vi "Solve General Linear Equations with SVD (DBL).vi"(8 "iteration":i32=2, 9 "relative tolerance":dbl, 10 "Known Vector":dbl[](array[numeric]), 11 "Input Matrix":T1) -> (0 "error":i32, 3 "Solution Vector":dbl[](array[numeric]))   [LabVIEW 2010, in "NI_AALPro.lvlib"]
uses:
  NI_AALPro.lvlib
  RealMatrix.ctl
  Real SVD Decomposition.vi
  Real Transpose Matrix.vi
  A x Vector.vi
  NI_AALBase.lvlib
  NI_Matrix.lvlib
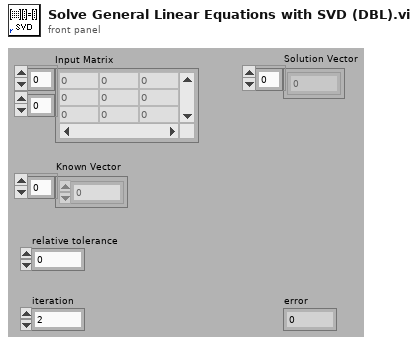
[diagram p1: front panel]
types:
  T1 = typedef "NI_Matrix.lvlib/RealMatrix.ctl" = dbl[][]
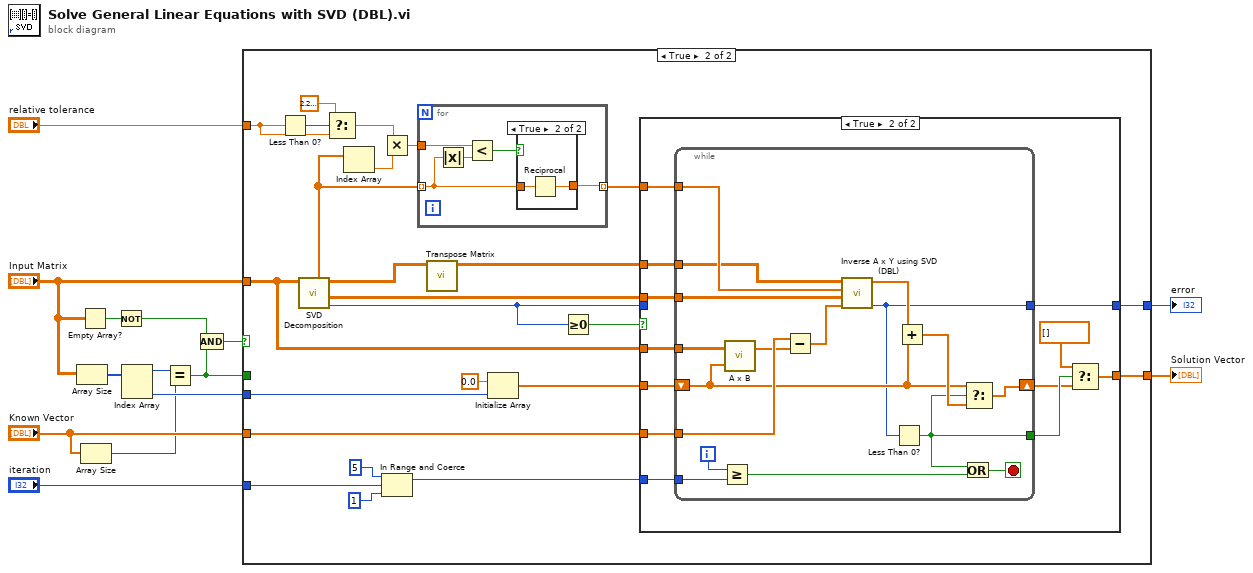
[diagram p0: block diagram]
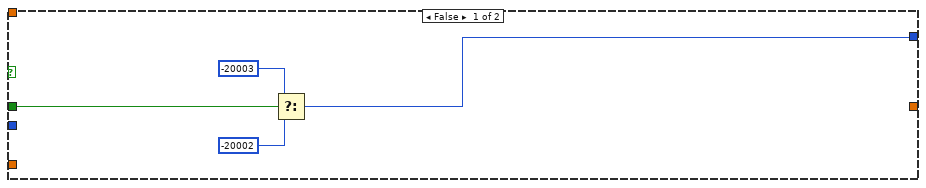
[diagram p2: hidden frame]
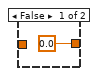
[diagram p4: hidden frame]
diagram:
  n1 = Array Size(array="Input Matrix") -> (size(s)=w12:i32[])
  n2 = Empty Array?(array="Input Matrix") -> (empty?=w6:bool)
  n3 = Array Size(array="Known Vector") -> (size(s)=w3:i32)
  n4 = Not(x=w6) -> (.not. x?=w5:bool)
  n5 = Index Array(array=w12) -> (element #1=w4:i32, element #2=w9:i32)  [unwired: 2 in]
  n6 = Equal?(x=w4, y=w3) -> (x = y?=w1:bool)
  n7 = Compound Arithmetic op=AND(w5, w1) -> (w2:bool)
  n8 = case shown="True" w2 {
    tunnel: "relative tolerance" -> [_ w41]
    tunnel: "Known Vector" -> [_ w31]
    tunnel: "iteration" -> [_ w30]
    tunnel: "Input Matrix" -> [_ w19]
    tunnel: w9 -> [_ w25]
    tunnel: [_ w22] -> w11
    tunnel: [w15 w21] -> w10
    tunnel: w1 -> [w18 _]
    frame False {
      n9 = Select(t=-20003, s=w18, f=-20002) -> (s? t:f=w15:i32)
    }
    frame True {
      n10 = Less Than 0?(x=w41) -> (x < 0?=w42:bool)
      n11 = call-poly "SVD Decomposition.vi"("A"=w19) -> ("error"=w20:i32, "Matrix V"=w34:T1, "Matrix U"=w35:T1, "Vector S"=w36:dbl[])  [unwired: 6 in, 1 out]
      n12 = Select(t=2.220446049250313e-16, s=w42, f=w41) -> (s? t:f=w39:dbl)
      n13 = Index Array(array=w36) -> (element=w38:dbl)  [unwired: 1 in]
      n14 = Multiply(x=w39, y=w38) -> (x*y=w37:dbl)
      n15 = In Range and Coerce(upper limit=5, x=w30, lower limit=1) -> (coerced(x)=w27:i32)  [unwired: 1 out]
      n16 = for {
        tunnel: w36 -> [w75] mode=indexing
        tunnel: w37 -> [w77]
        tunnel: [w73] -> w26 mode=indexing
        n17 = Absolute Value(x=w75) -> (abs(x)=w76:dbl)
        n18 = Less?(x=w77, y=w76) -> (x < y?=w74:bool)
        n19 = case shown="True" w74 {
          tunnel: w75 -> [_ w80]
          tunnel: [0.0 w79] -> w73
          frame False {
          }
          frame True {
            n20 = Reciprocal(x=w80) -> (1/x=w79:dbl)
          }
        }
      }
      n21 = call-poly "Transpose Matrix.vi"("Input Matrix"=w35) -> ("Matrix Transpose"=w33:T1)  [unwired: 9 in, 1 out]
      n22 = Initialize Array(0.0 ("element"), w25) -> (w23:dbl[])
      n23 = Greater Or Equal To 0?(x=w20) -> (x >= 0?=w32:bool)
      n24 = case shown="True" w32 {
        tunnel: w34 -> [_ w52]
        tunnel: w33 -> [_ w53]
        tunnel: w19 -> [_ w50]
        tunnel: w31 -> [_ w51]
        tunnel: w27 -> [_ w55]
        tunnel: w26 -> [_ w54]
        tunnel: w23 -> [_ w49]
        tunnel: [_ w44] -> w22
        tunnel: [w43 w48] -> w21
        tunnel: w20 -> [w43 _]
        frame False {
        }
        frame True {
          n25 = while {
            tunnel: w55 -> [w64]
            tunnel: w54 -> [w72]
            tunnel: w53 -> [w71]
            tunnel: w52 -> [w70]
            tunnel: w51 -> [w68]
            tunnel: w50 -> [w69]
            shift-right: [w59] -> w46
            shift-left: w49 -> [w58]
            tunnel: [w57] -> w48
            tunnel: [w56] -> w47
            i -> [w65]
            stop <- w62 stop-if-true
            n26 = Greater Or Equal?(x=w65, y=w64) -> (x >= y?=w63:bool)
            n27 = call-poly "A x B.vi"("Vector"=w58, "A"=w69) -> ("A x Vector"=w67:dbl[])  [unwired: 1 out]
            n28 = Subtract(x=w68, y=w67) -> (x-y=w66:dbl[])
            n29 = call "Inverse A x Y using SVD (DBL).vi"("Known Vector"=w66, "V"=w70, "1/S"=w72, "U*"=w71) -> ("error"=w57:i32, "Solution Vector"=w61:dbl[])  [unwired: 6 in]
            n30 = Less Than 0?(x=w57) -> (x < 0?=w56:bool)
            n31 = Add(x=w61, y=w58) -> (x+y=w60:dbl[])
            n32 = Or(x=w56, y=w63) -> (x .or. y?=w62:bool)
            n33 = Select(t=w58, s=w56, f=w60) -> (s? t:f=w59:dbl[])
          }
          n34 = Select(t=dbl[] [], s=w47, f=w46) -> (s? t:f=w44:dbl[])
        }
      }
    }
  }
  "Solution Vector" <- w11
  "error" <- w10
